vi "GetAttributes.vi"(0 "ClassReader in":refnum<class "ClassReader.lvclass">, 1 "OnlyGetReference":bool, 5 "error in (no error)":errorcluster) -> (14 "ClassReader out":refnum<class "ClassReader.lvclass">, 15 "ObjectAttributes":T1[](array[typedef])=[{"name"="MyU8", "type"=enum."UINT8", "dimension"=0, "typeName"="", "typePath"=path "", "visibility"=enum."Protected"}, {"name"="MyStrArray", "type"=enum."STRING", "dimension"=1, "typeName"="", "typePath"=path "", "visibility"=enum."Protected"}], 16 "ClassAttributes":T1[](array[typedef])=[{"name"="MyU8", "type"=enum."UINT8", "dimension"=0, "typeName"="", "typePath"=path "", "visibility"=enum."Protected"}, {"name"="MyStrArray", "type"=enum."STRING", "dimension"=1, "typeName"="", "typePath"=path "", "visibility"=enum."Protected"}], 17 "ObjectAttributeReference":refnum<vi>, 18 "ClassAttributeReference":refnum<vi>, 19 "error out":errorcluster)   [LabVIEW 2012, in "ClassReader.lvclass"]
uses:
  <resource>/Framework/Providers/Open_GDS/ClassProviders/Provider_BaseClassInterface/ClassReader_class/ClassReader.lvclass
  <resource>/Framework/Providers/Open_GDS/UML/ReversedEngineering/ReversedEngineering AttributeInfoType.ctl
  <resource>/Framework/Providers/Open_GDS/UML/ReversedEngineering/ReversedEngineering AttributeDataType.ctl
  <resource>/Framework/Providers/Open_GDS/UML/UMLEditor/UMLEditor_VisibilityType.ctl
  <resource>/Framework/Providers/Open_GDS/ClassProviders/Provider_BaseClassInterface/ClassReader_class/ClassReader.lvclass/ClassReader.ctl
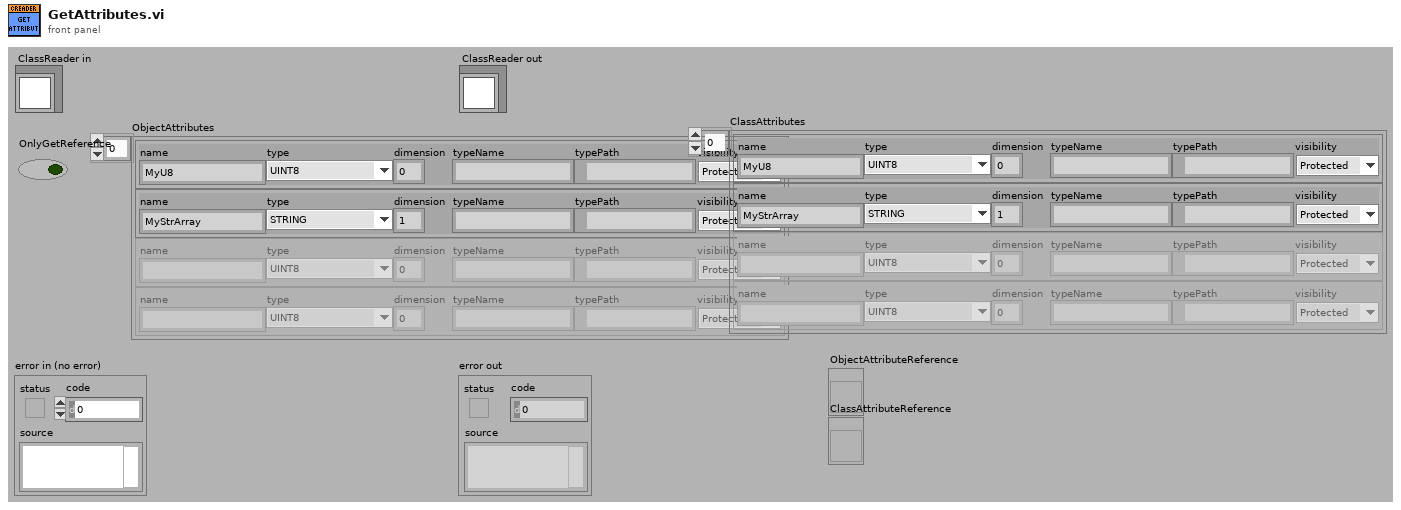
[diagram p1: front panel]
types:
  T1 = typedef "ReversedEngineering AttributeInfoType.ctl" = cluster{"name":string, "type":T2, "dimension":i32, "typeName":string, "typePath":path, "visibility":T3}
  T2 = typedef "ReversedEngineering AttributeDataType.ctl" = enum16{"UINT8", "INT8", "UINT16", "INT16", "UINT32", "INT32", "UINT64", "INT64", "SGL", "DBL", "EXT", "CSG", "CDB", "CXT", "TimeStamp", "STRING", "PATH", "BOOL", "ENUM", "RefNum", "VIRefNum", "ClassRefNum", "Cluster", "Variant", "TypeRef", "Waveform", "LabVIEW Object", "Other"}
  T3 = typedef "UMLEditor_VisibilityType.ctl" = enum16{"Public", "Private", "Protected"}
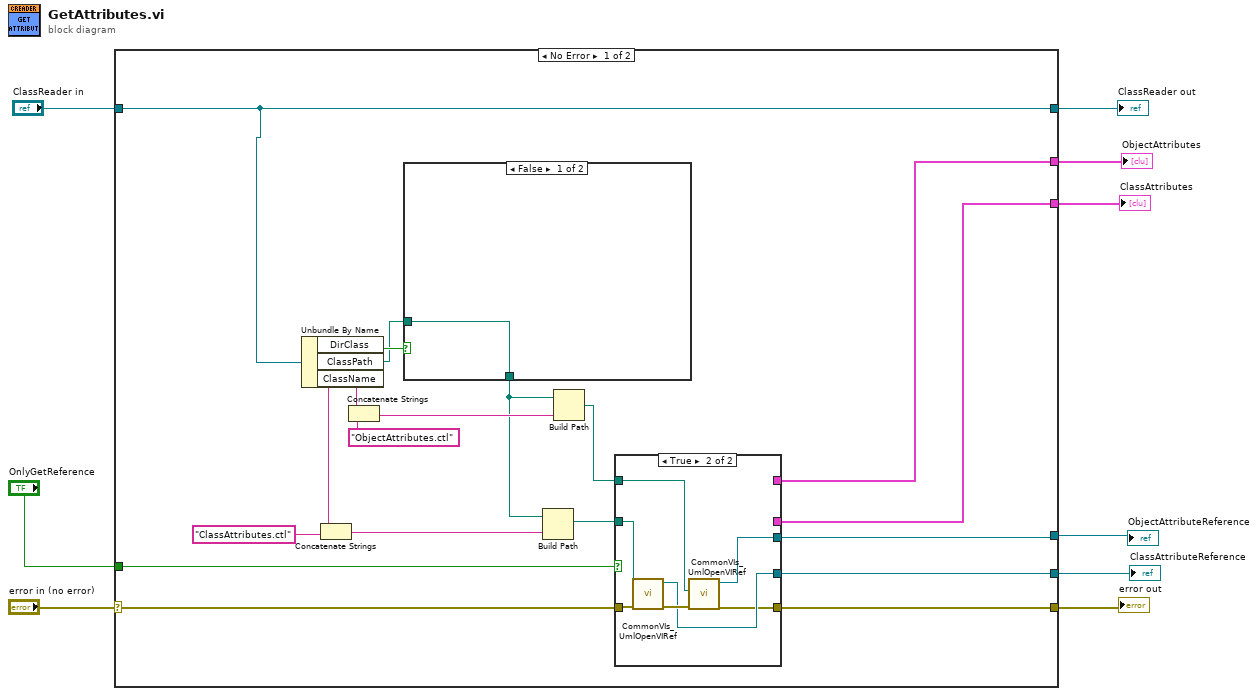
[diagram p0: block diagram]
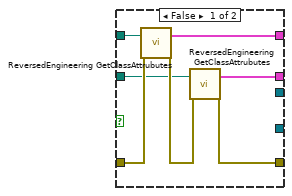
[diagram p2: hidden frame]
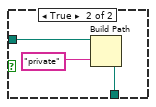
[diagram p3: hidden frame]
diagram:
  n1 = case shown="No Error" "error in (no error)" {
    selector: "error in (no error)" -> [w21 w47]
    tunnel: [w16 w47] -> w8
    tunnel: [w23 w46] -> w6
    tunnel: "ClassReader in" -> [w23 w46]
    tunnel: [w22 _] -> w5
    tunnel: [w15 _] -> w4
    tunnel: [w11 _] -> w3
    tunnel: [w10 _] -> w2
    tunnel: "OnlyGetReference" -> [w12 _]
    frame No Error {
      n2 = Unbundle By Name(w23) -> ("DirClass"=w25:bool, "ClassPath"=w24:path, "ClassName"=w19:string)
      n3 = Concatenate Strings(w19, "ClassAttributes.ctl" ("string")) -> (w17:string)
      n4 = Concatenate Strings(w19, "ObjectAttributes.ctl" ("string")) -> (w27:string)
      n5 = case shown="False" w25 {
        tunnel: w24 -> [w42 w44]
        tunnel: [w42 w45] -> w18
        frame False {
        }
        frame True {
          n6 = Build Path(base path=w44, name or relative path="private" ("element")) -> (appended path=w45:path)
        }
      }
      n7 = Build Path(base path=w18, name or relative path=w17) -> (appended path=w13:path)
      n8 = Build Path(base path=w18, name or relative path=w27) -> (appended path=w14:path)
      n9 = case shown="True" w12 {
        tunnel: [w34 _] -> w22
        tunnel: w21 -> [w33 w41]
        tunnel: [w31 w35] -> w16
        tunnel: [w30 _] -> w15
        tunnel: w14 -> [w29 w38]
        tunnel: w13 -> [w28 w40]
        tunnel: [_ w37] -> w11
        tunnel: [_ w36] -> w10
        frame False {
          n10 = call <resource>:"ReversedEngineering GetClassAttrubutes.vi"("Path(CtrlRenumf used if Path is empty)"=w29, "error in (no error)"=w33) -> ("attributeInfo"=w34:T1[], "error out"=w32:errorcluster)  [unwired: 15 in, 1 out]
          n11 = call <resource>:"ReversedEngineering GetClassAttrubutes.vi"("Path(CtrlRenumf used if Path is empty)"=w28, "error in (no error)"=w32) -> ("attributeInfo"=w30:T1[], "error out"=w31:errorcluster)  [unwired: 15 in, 1 out]
        }
        frame True {
          n12 = call <resource>:"CommonVIs_UmlOpenVIRef.vi"("error in"=w41, "ViPath/ViName"=w40) -> ("error out"=w39:errorcluster, "vi reference"=w36:refnum<vi>)  [unwired: 6 in, 2 out]
          n13 = call <resource>:"CommonVIs_UmlOpenVIRef.vi"("error in"=w39, "ViPath/ViName"=w38) -> ("error out"=w35:errorcluster, "vi reference"=w37:refnum<vi>)  [unwired: 6 in, 2 out]
        }
      }
    }
    frame Error {
    }
  }
  "error out" <- w8
  "ClassReader out" <- w6
  "ObjectAttributes" <- w5
  "ClassAttributes" <- w4
  "ObjectAttributeReference" <- w3
  "ClassAttributeReference" <- w2
